vi "Get Power Of 2.vi"(11 "Error Pointer in":refnum<class "Error Pointer.lvclass">) -> (2 "power of 2":i16, 3 "Error Pointer out":refnum<class "Error Pointer.lvclass">)   [LabVIEW 2017, in "DSF Core.lvlib" / "Error Pointer.lvclass"]
uses:
  Error Pointer.lvclass
  Error Pointer.lvclass/Error Pointer.ctl
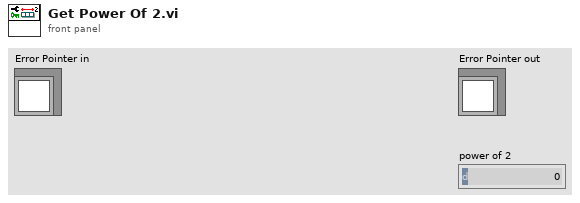
[diagram p1: front panel]
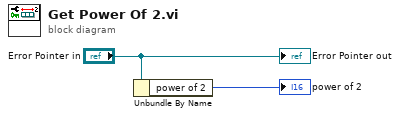
[diagram p0: block diagram]
diagram:
  n1 = Unbundle By Name("Error Pointer in") -> ("power of 2"=→"power of 2":i16)
  "Error Pointer out" <- "Error Pointer in"
